vi "shita_n__v1.vi"(9 "ƒÆ[n-1]":ext, 10 "R":ext, 11 "i[n]":ext) -> (3 "ƒÆ[n]":ext)   [LabVIEW 2020]
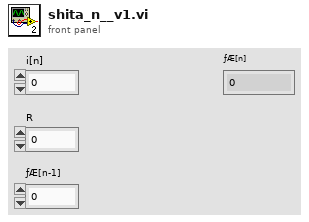
[diagram p1: front panel]
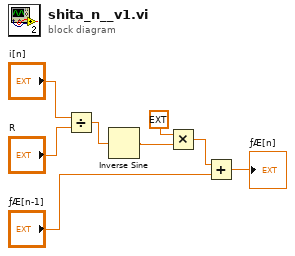
[diagram p0: block diagram]
diagram:
  n1 = Divide(x="i[n]", y="R") -> (x/y=w6:ext)
  n2 = Inverse Sine(1:w6) -> (0:w7:ext)
  n3 = Multiply(x=ext -2.0, y=w7) -> (x*y=w3:ext)
  n4 = Add(x=w3, y="ƒÆ[n-1]") -> (x+y=→"ƒÆ[n]":ext)
